vi "Test2-C.vi"(11 "Params":string[][](array[string])) -> ()   [LabVIEW 2017]
uses:
  C:/Users/Bendethic/Documents/LabVIEW Data/Projects/2018 Power Up/test-dependencies/Robot Project/Framework/Robot Global Data.vi
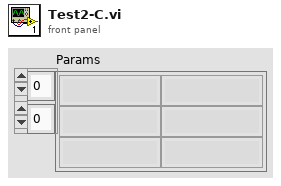
[diagram p1: front panel]
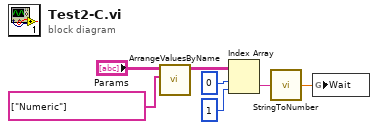
[diagram p0: block diagram]
diagram:
  n1 = call "ArrangeValuesByName.vi"("Names"=string[] ["Numeric"], "Names/Values in"="Params") -> ("Names/Values Out"=w5:string[][])  [unwired: 9 in]
  n2 = Index Array(array=w5, index (row)=0, index (col)=1) -> (element=w1:string)
  n3 = call "StringToNumber.vi"("String"=w1) -> ("Output"=w7:dbl)
  n4 = global write "Robot Global Data.vi" "Wait"(w7) -> ()
